vi "Create Function String (Integrate).vi"(8 "error in (no error)":errorcluster, 9 "Element (1: 1)":i32(ring)=1 items=["1"=1, "2"=2, "3"=3, "Sigma A"=4], 10 "Function (0: Time)":i32(ring) items=["Time", "WP", "WP+", "WP-", "q", "q+", "q-", "Math"], 11 "VISA resource name":refnum<visa-resource-name>) -> (0 "error out":errorcluster, 2 "Function String":string, 3 "VISA resource name out":refnum<visa-resource-name>)   [LabVIEW 2023, in "Yokogawa WT300 Series.lvlib"]
doc: "Create a integrate function string"
uses:
  Yokogawa WT300 Series.lvlib
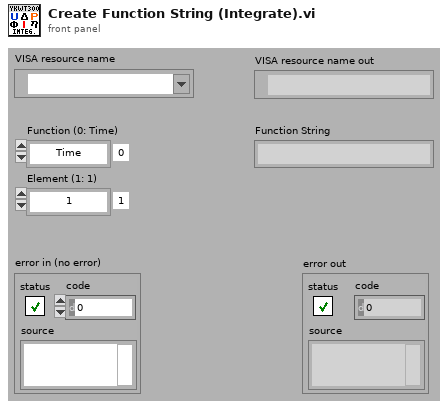
[diagram p1: front panel]
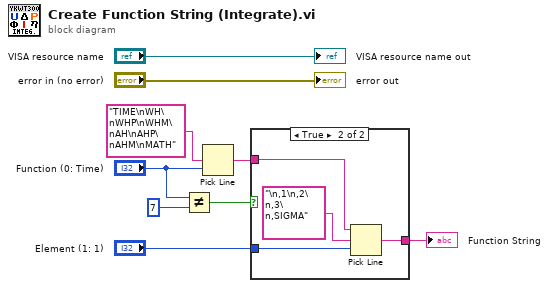
[diagram p0: block diagram]
diagram:
  n1 = Not Equal?(x="Function (0: Time)", y=7) -> (x != y?=w3:bool)
  n2 = Pick Line ("ライン選択")(multi-line string="TIME\nWH\nWHP\nWHM\nAH\nAHP\nAHM\nMATH" ("複数行文字列"), line index="Function (0: Time)") -> (output string=w4:string)  [unwired: 1 in]
  n3 = case shown="True" w3 {
    tunnel: "Element (1: 1)" -> [_ w14]
    tunnel: [w10 w13] -> w5
    tunnel: w4 -> [w10 w11]
    frame False {
      # "Select \"MATH\""
    }
    frame True {
      n4 = Pick Line ("ライン選択")(string ("")=w11, multi-line string="\n,1\n,2\n,3\n,SIGMA" ("複数行文字列"), line index=w14) -> (output string=w13:string)
    }
  }
  "Function String" <- w5
  "VISA resource name out" <- "VISA resource name"
  "error out" <- "error in (no error)"
